vi "FTP自动升级更新main.vi"() -> ()   [LabVIEW 2016, in "自动更新.lvlib"]
uses:
  <vilib>/FTP/NI_FTP.lvlib
panel:
  out "有新版本":bool
  out "最新版本获取进度":u8(slide) scale=0.0..100.0
  # "版本获取中，请稍后！"
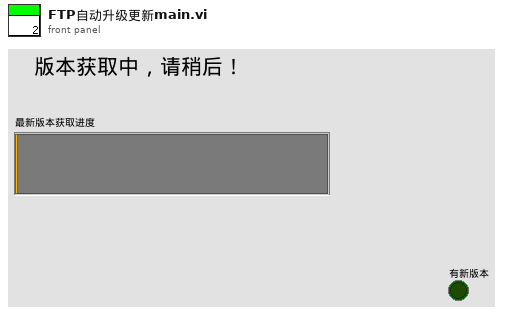
[diagram p1: front panel]
types:
  T1 = enum16{"get version information", "get success", "contact", "over"}
  T2 = cluster{"网络灯":bool, "接收中":bool, "已接收百分比":u8, "接收成功次数":dbl, "当前步骤":enum16{"init", "receivehead", "receivecontent", "receivesuccess", "over"}, "文件名":string, "error out":errorcluster}
  T3 = enum16{"open", "replace", "create", "open or create", "replace or create", "replace or create with confirmation"}
  T4 = cluster{"主机":string, "用户":string, "密码":string, "远程路径":string, "下载文件名":string, "软件版本":string}
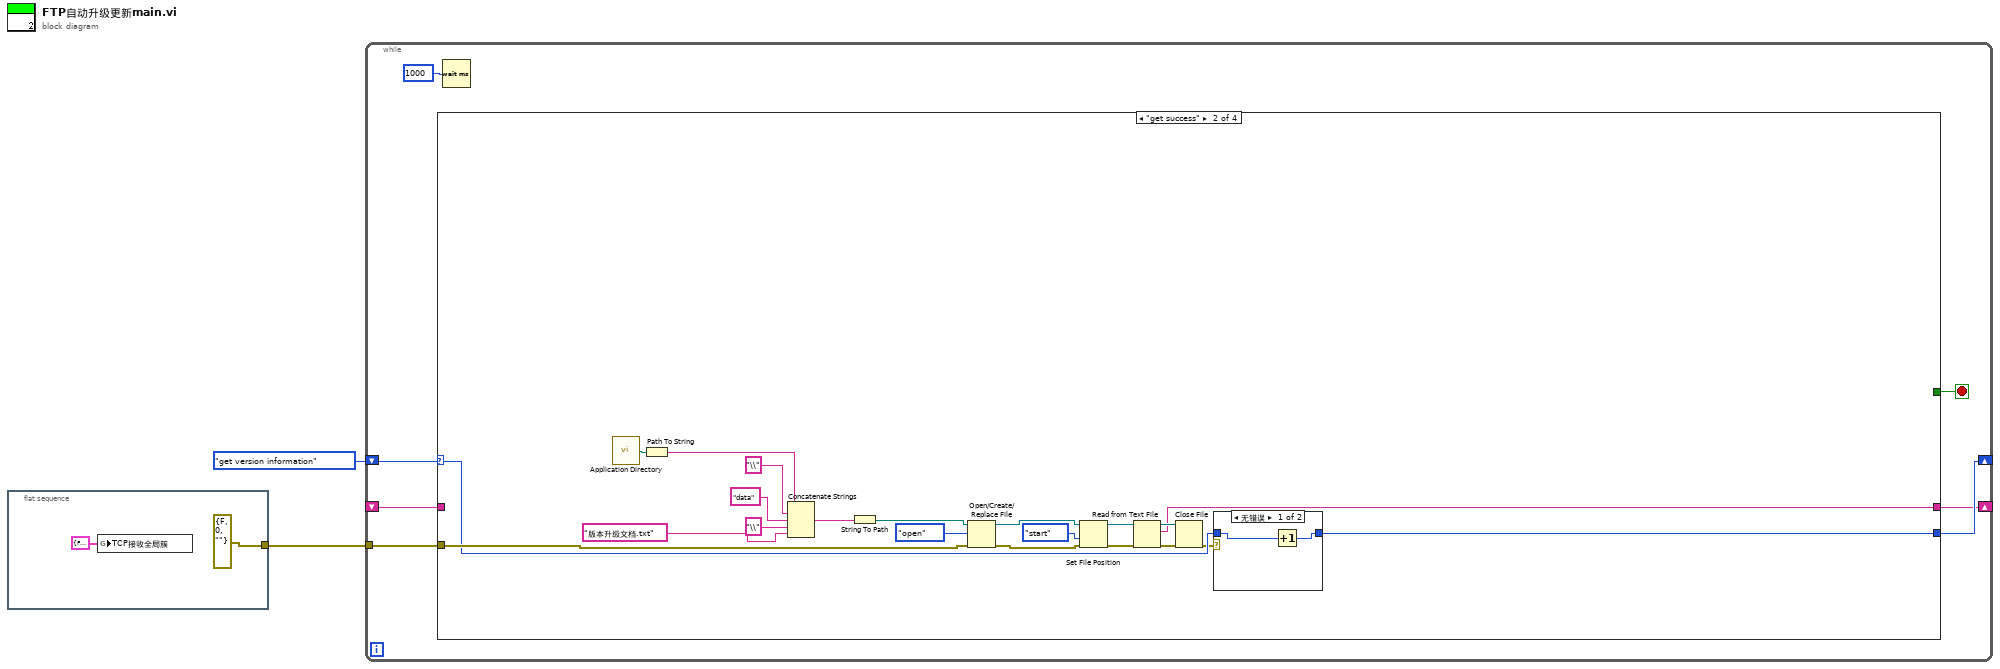
[diagram p0: block diagram]
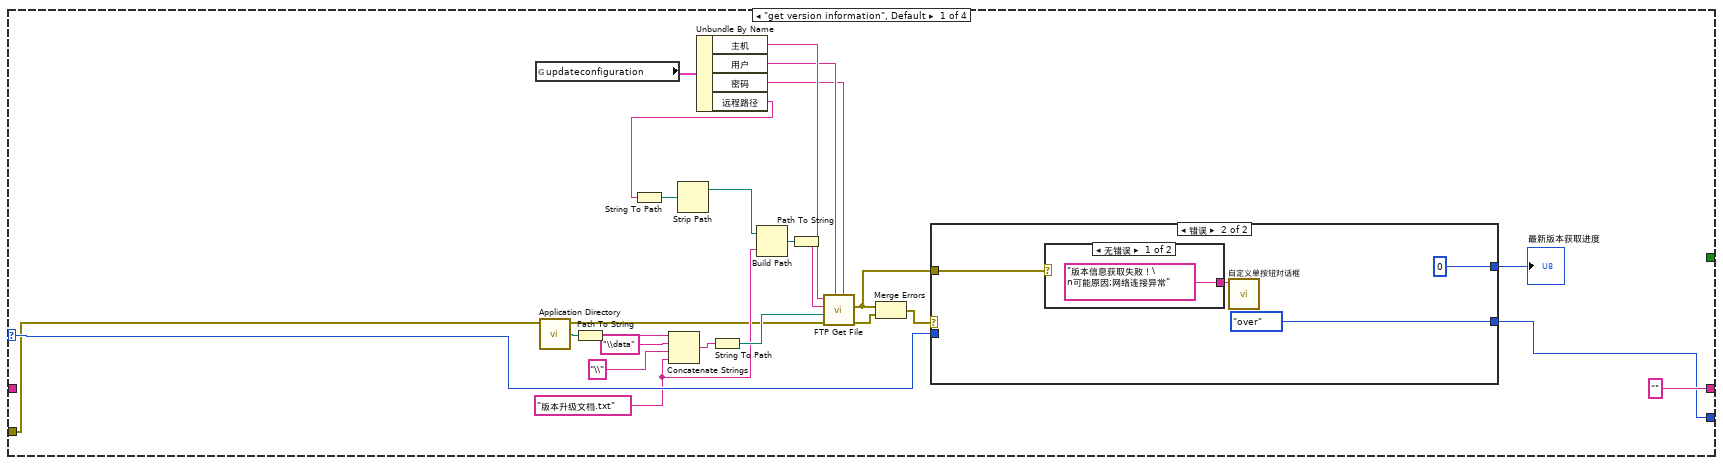
[diagram p2: hidden frame]
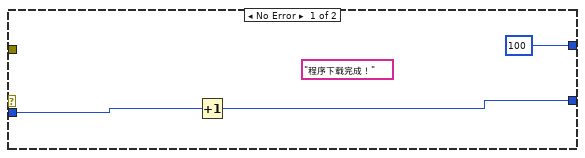
[diagram p3: hidden frame]
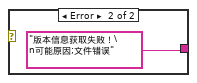
[diagram p4: hidden frame]
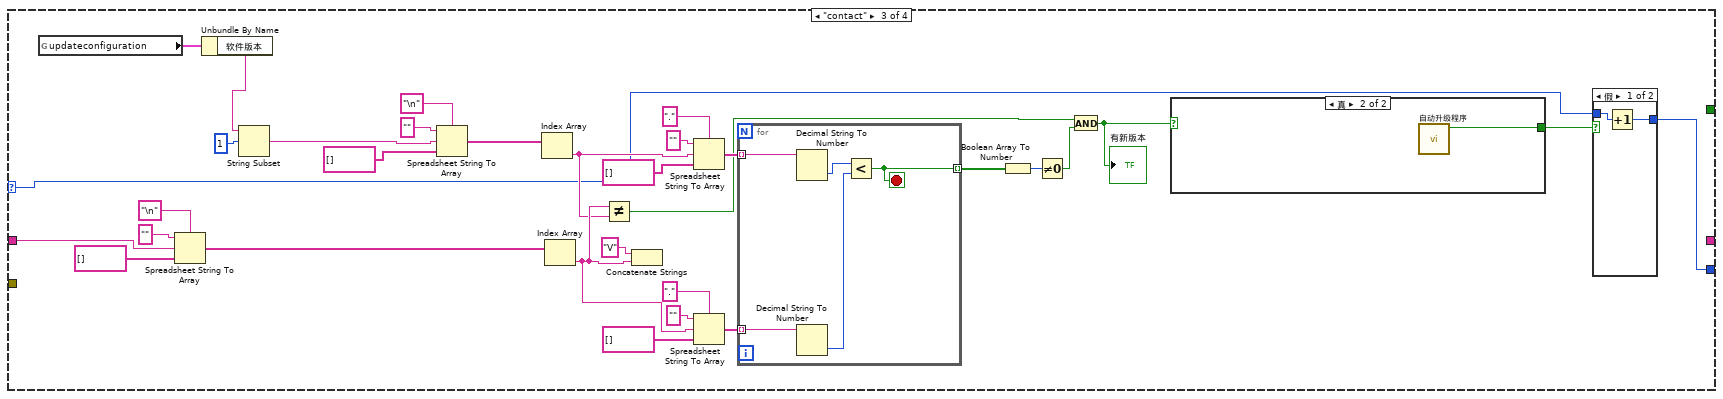
[diagram p6: hidden frame]
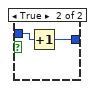
[diagram p7: hidden frame]
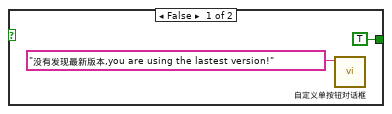
[diagram p8: hidden frame]
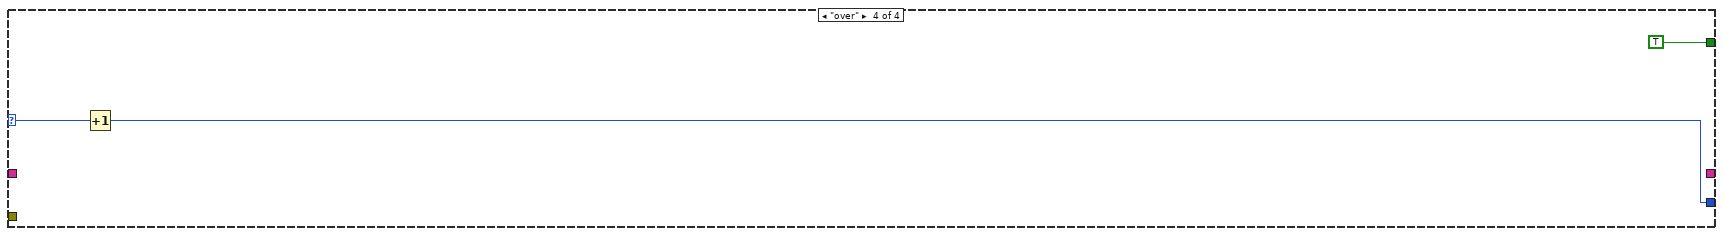
[diagram p9: hidden frame]
diagram:
  n1 = flat-sequence {
    tunnel: [errorcluster {"status"=FALSE, "code"=0, "source"=""} ("错误常量")] -> w1
    frame #0 {
      n2 = global write "全局变量1.vi" "TCP接收全局簇"(T2 {"网络灯"=FALSE, "接收中"=FALSE, "已接收百分比"=0, "接收成功次数"=0.0, "当前步骤"=enum."init", "文件名"="", "error out"={"status"=FALSE, "code"=0, "source"=""}} ("TCP接收全局簇")) -> ()
    }
  }
  n3 = while {
    shift-right: [w9] -> _
    shift-left: T1."get version information" -> [w10]
    tunnel: w1 -> [w8]
    shift-right: [w7] -> _
    shift-left: _ -> [w6]
    stop <- w5 stop-if-true
    n4 = case shown="\"get success\"" w10 {
      selector: w10 -> [w25 w52 w72 w114]
      tunnel: [w24 w51 w71 w113] -> w9
      tunnel: w8 -> [w12 w53 _ _]
      tunnel: ["" w45 _ _] -> w7
      tunnel: w6 -> [_ _ w75 _]
      tunnel: [_ _ _ TRUE] -> w5
      frame "get version information", Default {
        w15 = "版本升级文档.txt"
        n5 = global read "update全局.vi" "updateconfiguration"() -> (w23:T4)
        n6 = call <vilib>:"Application Directory.vi"() -> ("Application Directory"=w32:path)
        n7 = Path To String(path=w32) -> (string=w34:string)
        n8 = Concatenate Strings(w34, "\\data" ("字符串"), "\\" ("字符串"), w15) -> (w31:string)
        n9 = Unbundle By Name(w23) -> ("主机"=w22:string, "用户"=w21:string, "密码"=w20:string, "远程路径"=w16:string)
        n10 = String To Path(string=w16) -> (path=w18:path)
        n11 = Strip Path(path=w18) -> (stripped path=w17:path)  [unwired: 1 out]
        n12 = String To Path(string=w31) -> (path=w30:path)
        n13 = Build Path(base path=w17, name or relative path=w15) -> (appended path=w14:path)
        n14 = Path To String(path=w14) -> (string=w13:string)
        n15 = call <vilib>:"FTP Get File.vi"("password"=w20, "user"=w21, "error in (no error)"=w12, "local path"=w30, "remote path"=w13, "host"=w22) -> ("error out"=w29:errorcluster, "file error"=w27:errorcluster)  [unwired: 4 in]
        n16 = Merge Errors(w27, w29) -> (w28:errorcluster)
        n17 = case shown="错误" w28 {
          tunnel: w27 -> [_ w41]
          tunnel: [u8 100 ("y") u8 0 ("y")] -> w26
          tunnel: [w37 T1."over"] -> w24
          tunnel: w25 -> [w36 _]
          frame No Error {
            (unwired) "程序下载完成！"
            n18 = Increment(x=w36) -> (x+1=w37:T1)
          }
          frame Error {
            n19 = case shown="无错误" w41 {
              tunnel: ["版本信息获取失败！\n可能原因;网络连接异常" "版本信息获取失败！\n可能原因;文件错误"] -> w42
              frame No Error {
              }
              frame Error {
              }
            }
            n20 = call "自定义单按钮对话框.vi"("消息"=w42) -> ()  [unwired: 11 in]
          }
        }
        "最新版本获取进度" <- w26
      }
      frame "get success" {
        n21 = call <vilib>:"Application Directory.vi"() -> ("Application Directory"=w58:path)
        n22 = Path To String(path=w58) -> (string=w61:string)
        n23 = Concatenate Strings(w61, "\\" ("字符串"), "data" ("字符串"), "\\" ("字符串"), "版本升级文档.txt" ("字符串")) -> (w55:string)
        n24 = String To Path(string=w55) -> (path=w54:path)
        n25 = Open/Create/Replace File(file path (use dialog)=w54, error in=w53, operation (0:open)=T3."open" ("操作(0:open)")) -> (refnum out=w64:refnum<file>, error out=w63:errorcluster)  [unwired: 3 in, 1 out]
        n26 = Set File Position(refnum=w64, from (0:start)=enum16{"start", "end", "current"}."start" ("自（0:起始）"), error in=w63) -> (refnum out=w49:refnum<file>, error out=w48:errorcluster)  [unwired: 1 in]
        n27 = Read from Text File(file (use dialog)=w49, error in=w48) -> (refnum out=w50:refnum<file>, text=w45:string, error out=w47:errorcluster)  [unwired: 2 in, 1 out]
        n28 = Close File(refnum=w50, error in=w47) -> (error out=w46:errorcluster)  [unwired: 1 out]
        n29 = case shown="无错误" w46 {
          tunnel: w52 -> [w67 w68]
          tunnel: [w66 w68] -> w51
          frame No Error {
            n30 = Increment(x=w67) -> (x+1=w66:T1)
          }
          frame Error {
          }
        }
      }
      frame "contact" {
        n31 = global read "update全局.vi" "updateconfiguration"() -> (w70:T4)
        n32 = Spreadsheet String To Array(delimiter (Tab)="\n" ("分隔符(Tab)"), format string="" ("格式字符串"), spreadsheet string=w75, array type (2D Dbl)=string[] []) -> (array=w96:string[])
        n33 = Unbundle By Name(w70) -> ("软件版本"=w69:string)
        n34 = String Subset(string=w69, offset (0)=1 ("偏移量(0)")) -> (substring=w88:string)  [unwired: 1 in]
        n35 = Spreadsheet String To Array(delimiter (Tab)="\n" ("分隔符(Tab)"), format string="" ("格式字符串"), spreadsheet string=w88, array type (2D Dbl)=string[] []) -> (array=w87:string[])
        n36 = Index Array(array=w87) -> (element=w78:string)  [unwired: 1 in]
        n37 = Index Array(array=w96) -> (element=w79:string)  [unwired: 1 in]
        n38 = Not Equal?(x=w79, y=w78) -> (x != y?=w76:bool)
        n39 = Concatenate Strings("V" ("字符串"), w79) -> ()  [unwired: 1 out]
        n40 = Spreadsheet String To Array(delimiter (Tab)="." ("分隔符(Tab)"), format string="" ("格式字符串"), spreadsheet string=w78, array type (2D Dbl)=string[] []) -> (array=w82:string[])
        n41 = Spreadsheet String To Array(delimiter (Tab)="." ("分隔符(Tab)"), format string="" ("格式字符串"), spreadsheet string=w79, array type (2D Dbl)=string[] []) -> (array=w83:string[])
        n42 = for {
          tunnel: w83 -> [w110] mode=indexing
          tunnel: w82 -> [w112] mode=indexing
          tunnel: [w111] -> w81 mode=indexing
          stop <- w111 stop-if-true
          n43 = Decimal String To Number(string=w112) -> (number=w109:i32)  [unwired: 2 in, 1 out]
          n44 = Decimal String To Number(string=w110) -> (number=w108:i32)  [unwired: 2 in, 1 out]
          n45 = Less?(x=w109, y=w108) -> (x < y?=w111:bool)
        }
        n46 = Boolean Array To Number(Boolean array=w81) -> (number=w80:u32)
        n47 = Not Equal To 0?(x=w80) -> (x != 0?=w77:bool)
        n48 = And(x=w76, y=w77) -> (x .and. y?=w74:bool)
        "有新版本" <- w74
        n49 = case shown="真" w74 {
          tunnel: [TRUE ("确定") w107] -> w73
          frame False {
            n50 = call "自定义单按钮对话框.vi"("消息"="没有发现最新版本,you are using the lastest version!") -> ()  [unwired: 11 in]
          }
          frame True {
            n51 = call "自动升级程序.vi"() -> ("确定"=w107:bool)  [unwired: 10 in, 1 out]
          }
        }
        n52 = case shown="假" w73 {
          tunnel: w72 -> [w102 w104]
          tunnel: [w101 w103] -> w71
          frame False {
            n53 = Increment(x=w102) -> (x+1=w101:T1)
          }
          frame True {
            n54 = Increment(x=w104) -> (x+1=w103:T1)
          }
        }
      }
      frame "over" {
        n55 = Increment(x=w114) -> (x+1=w113:T1)
      }
    }
    n56 = Wait (ms)(milliseconds to wait=u32 1000 ("等待时间（毫秒）")) -> ()  [unwired: 1 out]
  }
